vi "VideoWriter Dispose.vi"(8 "error in (no error)":errorcluster, 11 "VideoWriter in":refnum<class "VideoWriter.lvclass">) -> (0 "error out":errorcluster)   [LabVIEW 2020, in "OpenLvVision_OpenCv.lvlib" / "VideoWriter.lvclass"]
doc: "Closes the reference and triggers cleanup of the associated C++ object, releasing system resources.\nYou must call this VI when you are finished using the object reference to prevent memory leaks!"
uses:
  VideoWriter.lvclass
  _LvHelpers/EdvrObject/EdvrObject.lvclass
  C:/Users/lukas/Downloads/OpenLvVision_OpenCv/SourceCode/LabView/OpenLvVision_OpenCv/_LvHelpers/EdvrObject/EdvrObject.lvclass
  C:/Users/lukas/Downloads/OpenLvVision_OpenCv/SourceCode/LabView/OpenLvVision_OpenCv/VideoIO/VideoWriter/VideoWriter.lvclass
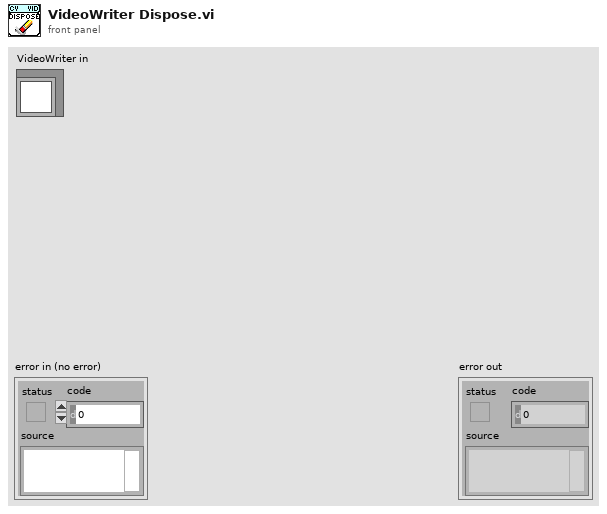
[diagram p1: front panel]
types:
  T1 = typedef "OpenLvVision_OpenCv.lvlib/EdvrObject.lvclass/Edvr.ctl" = refnum<data-value>
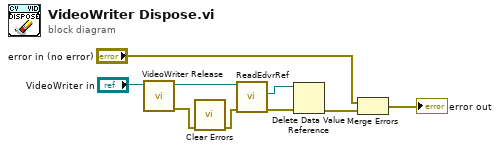
[diagram p0: block diagram]
diagram:
  n1 = call "VideoWriter Release.vi"("VideoWriter in"="VideoWriter in") -> ("error out"=w4:errorcluster, "VideoWriter out"=w6:refnum<class "VideoWriter.lvclass">)  [unwired: 9 in]
  n2 = call <vilib>:"Clear Errors.vi"("error in (no error)"=w4) -> ("error out"=w5:errorcluster)  [unwired: 5 in, 1 out]
  n3 = call "ReadEdvrRef.vi"("error in (no error)"=w5, "EdvrObject in"=w6) -> ("error out"=w9:errorcluster, "Edvr"=w8:T1)  [unwired: 7 in, 1 out]
  n4 = Delete Data Value Reference(data value reference=w8, error in=w9) -> (error out=w7:errorcluster)  [unwired: 1 out]
  n5 = Merge Errors("error in (no error)", w7) -> (→"error out":errorcluster)
